vi "SVT Crest Factor (N Ch).vi"(6 "restart averaging (F)":bool, 8 "error in (no error)":errorcluster, 11 "scaled signals [EU]":waveform(dbl)[](array[waveform])) -> (0 "error out":errorcluster, 1 "RMS levels [EU rms]":dbl[](array[numeric]) format="%.2f", 2 "peak levels [EU]":dbl[](array[numeric]) format="%.2f", 3 "crest factors":dbl[](array[numeric]) format="%.2f")   [LabVIEW 2017]
doc: "Computes the crest factor, peak level, and RMS level of <B>scaled signal [EU]</B> or <B>even angle signal [EU]</B>. You can use this polymorphic VI to compute the crest factor for a single channel or for N channels, or for a single channel or N channels of resampled data. The data type you wire to the <B>scaled signal [EU]</B> or <B>even angle signal [EU]</B> input determines the polymorphic instance to use."
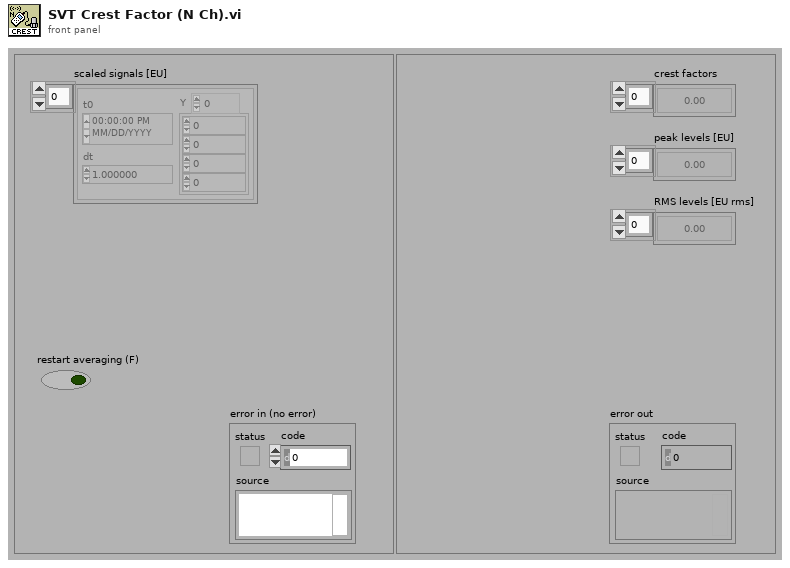
[diagram p1: front panel]
types:
  T1 = enum16{"RMS", "Running RMS", "Exp avg  ", "Dec exp avg ", "Peak", "Crest"}
  T2 = enum16{"Reset filter", "Restart averaging", "Continue processing"}
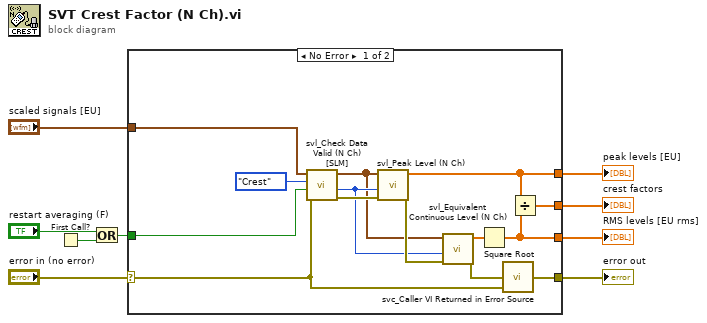
[diagram p0: block diagram]
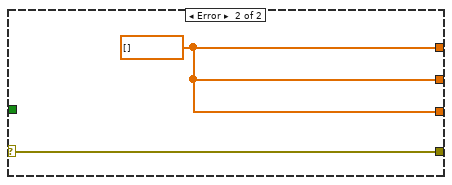
[diagram p2: hidden frame]
diagram:
  n1 = First Call?() -> (First Call?: T/F=w4:bool)
  n2 = Or(x="restart averaging (F)", y=w4) -> (x .or. y?=w2:bool)
  n3 = case shown="No Error" "error in (no error)" {
    selector: "error in (no error)" -> [w10 w25]
    tunnel: "scaled signals [EU]" -> [w12 _]
    tunnel: [w18 w25] -> w8
    tunnel: [w14 w24] -> w7
    tunnel: [w21 w24] -> w6
    tunnel: [w20 w24] -> w5
    tunnel: w2 -> [w16 _]
    frame No Error {
      n4 = call <vilib>:"svl_Check Data Valid (N Ch) [SLM].vi"("error in (no error)"=w10, "restart averaging (F)"=w16, "level analysis"=T1."Crest" ("Level Analysis"), "scaled signals [EU]"=w12) -> ("error out"=w17:errorcluster, "processing state"=w15:T2, "dup scaled signals [EU]"=w11:waveform(dbl)[])  [unwired: 5 in]
      n5 = call <vilib>:"svl_Peak Level (N Ch).vi"("error in (no error)"=w17, "processing state"=w15, "scaled signals [EU]"=w11) -> ("error out"=w19:errorcluster, "peak levels"=w14:dbl[])  [unwired: 7 in]
      n6 = call <vilib>:"svl_Equivalent Continuous Level (N Ch).vi"("error in (no error)"=w19, "processing state"=w15, "scaled signals [EU]"=w11) -> ("error out"=w23:errorcluster, "equivalent continuous levels [EU^2 rms]"=w22:dbl[])  [unwired: 7 in]
      n7 = Square Root(x=w22) -> (sqrt(x)=w21:dbl[])
      n8 = call <vilib>:"svc_Caller VI Returned in Error Source.vi"("warning input to caller"=w10, "error in (no error)"=w23) -> ("error out"=w18:errorcluster)  [unwired: 3 in]
      n9 = Divide(x=w14, y=w21) -> (x/y=w20:dbl[])
    }
    frame Error {
      w24 = dbl[] []
    }
  }
  "RMS levels [EU rms]" <- w6
  "error out" <- w8
  "peak levels [EU]" <- w7
  "crest factors" <- w5
